vi "C843Config.vi"(1 "Axes to Move":string[](array[string]), 2 "Initialisation OK Refnum":refnum<vi>, 3 "All Axes? Refnum":refnum<vi>, 4 "Stage names Input Refnum":refnum<vi>, 5 "Identification Refnum":refnum<vi>, 6 "Connected Axes Refnum":refnum<vi>, 7 "Position Refnum":refnum<vi>, 10 "+/- movement range Refnum":refnum<vi>, 11 "Error Out Refnum":refnum<vi>, 12 "LED status Refnum":refnum<vi>, 13 "Etat moteurs Refnum":refnum<vi>) -> ()   [LabVIEW 2013]
panel:
  in  "LED status Refnum 2":refnum<vi>
  out "Identification":string
  out "Conn. \nAxes":string[](array[string])
  out "Position":dbl[](array[numeric]) format="%.6f"
  out "+/- movement\nrange":dbl[](array[numeric]) format="%.6f"
  out "Stage names input":string[](array[string])
  out "All Axes?":bool
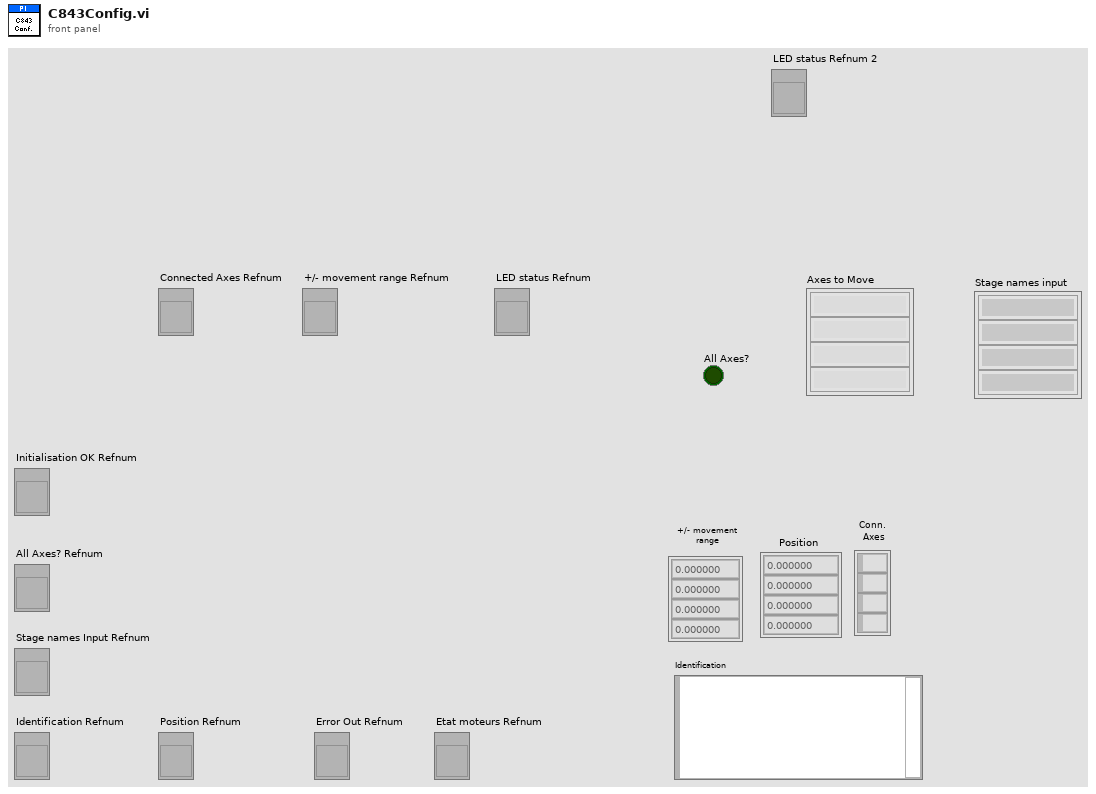
[diagram p1: front panel]
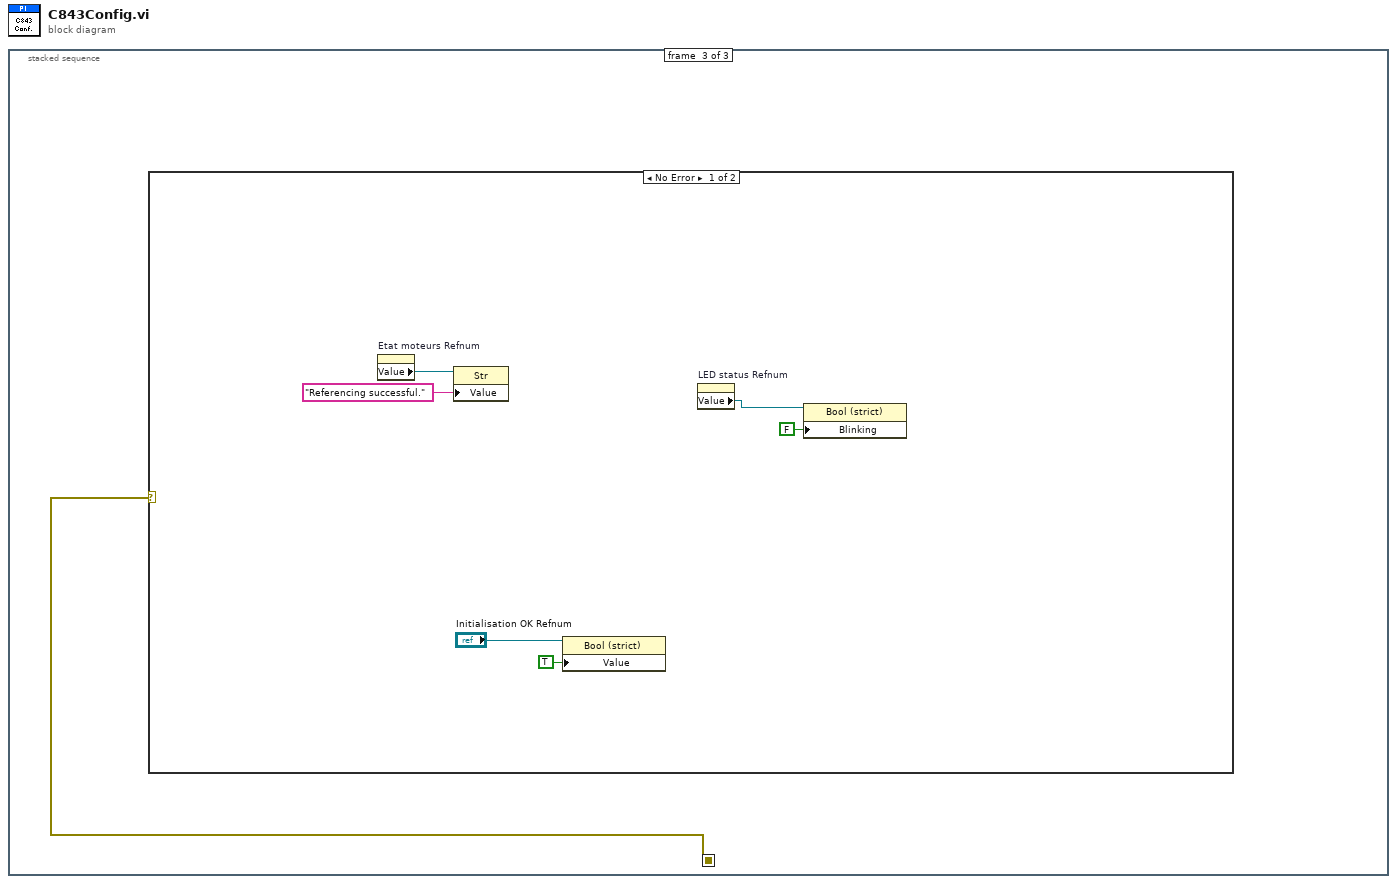
[diagram p0: block diagram]
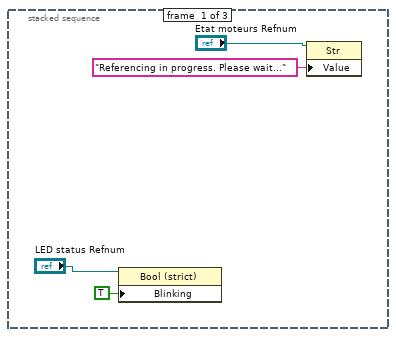
[diagram p2: hidden frame]
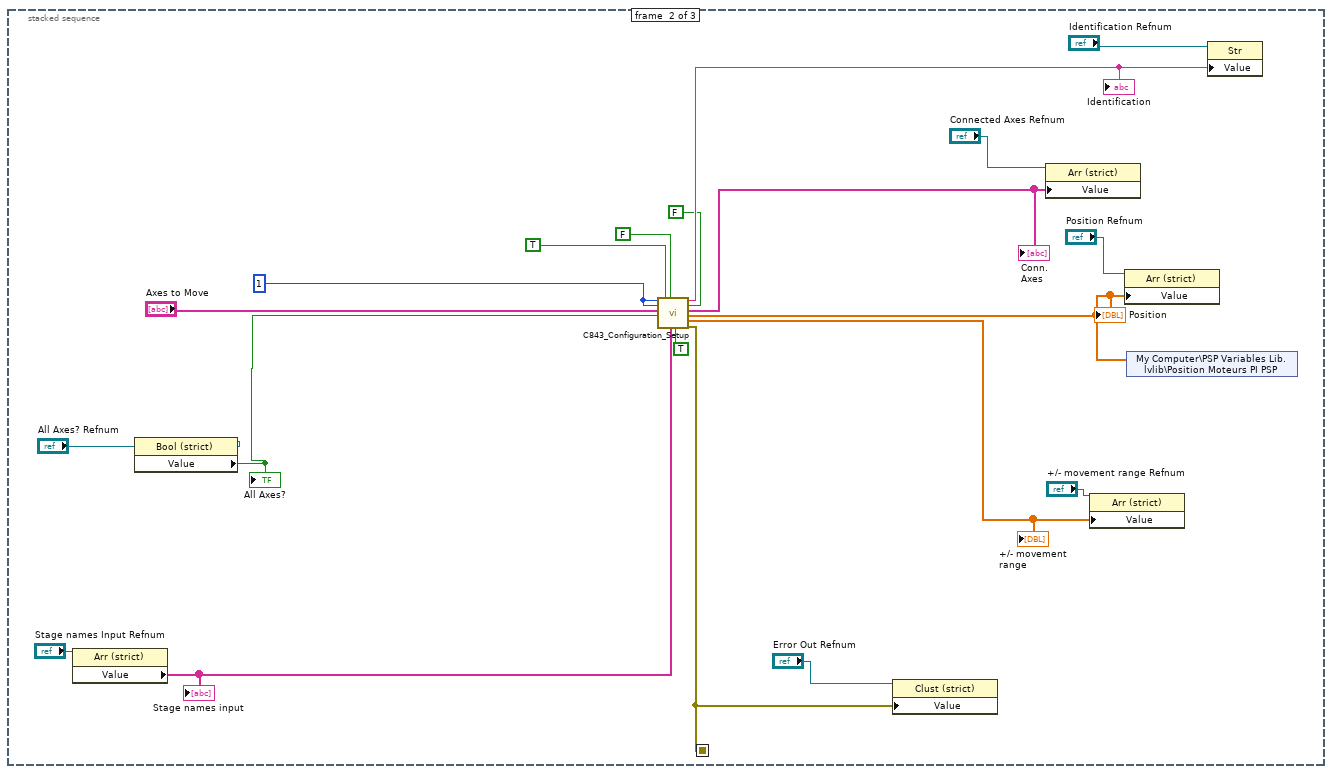
[diagram p3: hidden frame]
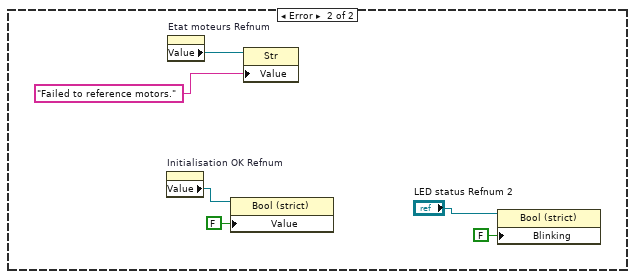
[diagram p4: hidden frame]
diagram:
  n1 = stacked-sequence {
    seq-local: [_ w13 _] -> [_ _ w25]
    frame #0 {
      n2 = property class="Bool (strict)"(reference="LED status Refnum", "Blinking"=TRUE) -> ()  [unwired: 1 in, 2 out]
      n3 = property class="Str"(reference="Etat moteurs Refnum", "Value"="Referencing in progress. Please wait...") -> ()  [unwired: 1 in, 2 out]
    }
    frame #1 {
      w10 = 1 ("System no.")
      n4 = property class="Arr (strict)"(reference="Stage names Input Refnum") -> ("Value"=w9:string[])  [unwired: 1 in, 2 out]
      "Stage names input" <- w9
      n5 = property class="Bool (strict)"(reference="All Axes? Refnum") -> ("Value"=w24:bool)  [unwired: 1 in, 2 out]
      "All Axes?" <- w24
      n6 = call "C843_Configuration_Setup.vi"("System no."=w10, "C-843 Board No."=w10, "Axes to move"="Axes to Move", "All axes?"=w24, "C-843 version"=TRUE, "Use dialog to define\nconnected stages?"=FALSE ("Use dialog to define\nconnected stages?"), "Stage names input"=w9, "Define home?"=TRUE, "Move to middle?"=FALSE) -> ("Identification"=w23:string, "Conn. \nAxes"=w22:string[], "Position"=w12:dbl[], "+/- movement\nrange"=w21:dbl[], "error out"=w13:errorcluster)  [unwired: 6 in]
      "+/- movement\nrange" <- w21
      "Position" <- w12
      "Conn. \nAxes" <- w22
      "Identification" <- w23
      n7 = property class="Clust (strict)"(reference="Error Out Refnum", "Value"=w13) -> ()  [unwired: 1 in, 2 out]
      n8 = property class="Arr (strict)"(reference="Connected Axes Refnum", "Value"=w22) -> ()  [unwired: 1 in, 2 out]
      n9 = property class="Arr (strict)"(reference="+/- movement range Refnum", "Value"=w21) -> ()  [unwired: 1 in, 2 out]
      n10 = property class="Arr (strict)"(reference="Position Refnum", "Value"=w12) -> ()  [unwired: 1 in, 2 out]
      n11 = shared-variable "My Computer\\PSP Variables Lib.lvlib\\Position Moteurs PI PSP"(w12) -> ()  [unwired: 1 in, 1 out]
      n12 = property class="Str"(reference="Identification Refnum", "Value"=w23) -> ()  [unwired: 1 in, 2 out]
    }
    frame #2 {
      n13 = case shown="No Error" w25 {
        frame No Error {
          n14 = property on="Etat moteurs Refnum" class="LVObjRef (strict)"() -> ("Value"=w31:refnum<vi>)  [unwired: 2 in, 2 out]
          n15 = property class="Str"(reference=w31, "Value"="Referencing successful.") -> ()  [unwired: 1 in, 2 out]
          n16 = property class="Bool (strict)"(reference="Initialisation OK Refnum", "Value"=TRUE) -> ()  [unwired: 1 in, 2 out]
          n17 = property on="LED status Refnum" class="LVObjRef (strict)"() -> ("Value"=w27:refnum<vi>)  [unwired: 2 in, 2 out]
          n18 = property class="Bool (strict)"(reference=w27, "Blinking"=FALSE) -> ()  [unwired: 1 in, 2 out]
        }
        frame Error {
          n19 = property on="Initialisation OK Refnum" class="LVObjRef (strict)"() -> ("Value"=w35:refnum<vi>)  [unwired: 2 in, 2 out]
          n20 = property on="Etat moteurs Refnum" class="LVObjRef (strict)"() -> ("Value"=w37:refnum<vi>)  [unwired: 2 in, 2 out]
          n21 = property class="Bool (strict)"(reference=w35, "Value"=FALSE) -> ()  [unwired: 1 in, 2 out]
          n22 = property class="Str"(reference=w37, "Value"="Failed to reference motors.") -> ()  [unwired: 1 in, 2 out]
          n23 = property class="Bool (strict)"(reference="LED status Refnum 2", "Blinking"=FALSE) -> ()  [unwired: 1 in, 2 out]
        }
      }
    }
  }
